vi "Close.vi"(8 "error in (no error)":errorcluster, 11 "navX - SERIAL in":refnum<class "navX - SERIAL.lvclass">) -> (0 "error out":errorcluster, 3 "navX - SERIAL out":refnum<class "navX - SERIAL.lvclass">)   [LabVIEW 2015, in "navX Library v3.lvlib" / "navX - SERIAL.lvclass"]
uses:
  navX - SERIAL.lvclass
  navX - SERIAL.lvclass/navX - SERIAL.ctl
  navX - Base/navX - Base.lvclass
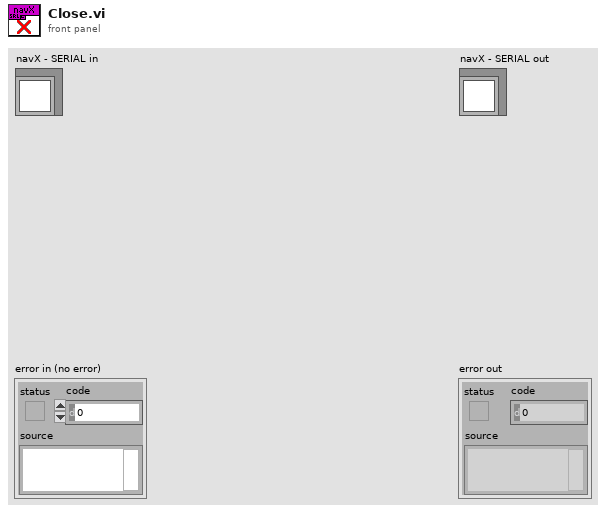
[diagram p1: front panel]
types:
  T1 = typedef "WPI_SerialPortRef.ctl" = cluster{"DevStatus":errorcluster, "Serial Port Name":refnum<visa-resource-name>}
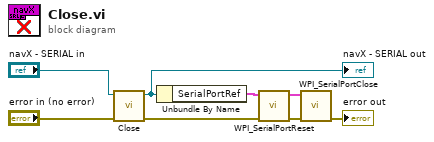
[diagram p0: block diagram]
diagram:
  n1 = call-parent "Close.vi"("error in (no error)"="error in (no error)", "navX - Base in"="navX - SERIAL in") -> ("error out"=w8:errorcluster, "navX - Base out"=w2:refnum<class "navX - SERIAL.lvclass">)  [unwired: 8 in]
  "navX - SERIAL out" <- w2
  n2 = Unbundle By Name(w2) -> ("SerialPortRef"=w1:T1)
  n3 = call <vilib>:"WPI_SerialPortReset.vi"("error in (no error)"=w8, "SerialPortRef"=w1) -> ("error out"=w5:errorcluster, "SerialPortRef"=w3:T1)  [unwired: 8 in]
  n4 = call <vilib>:"WPI_SerialPortClose.vi"("error in (no error)"=w5, "SerialPortRef"=w3) -> ("error out"=→"error out":errorcluster)  [unwired: 9 in]
